vi "Add Test Suite - Without Id - Reports Error.vi"() -> ()   [LabVIEW 2013, in "JUnit XML Tests.lvlib" / "Test Suites.lvlib"]
uses:
  Test Suites.lvlib
  JUnit XML/Test Suite/Test Suite.lvclass/Test Suite.ctl
  JUnit XML/Test Suite/Write Timestamp.vi
  <vilib>/addons/_JKI Toolkits/Caraya/classes/Assert/Assert Error.vi
  <vilib>/addons/_JKI Toolkits/Caraya/classes/Test/Test.lvclass
  <vilib>/addons/_JKI Toolkits/Caraya/classes/Assert/Assert.lvclass
  JUnit XML/Test Suites/Test Suites.lvclass
  JUnit XML/Test Suite/Test Suite.lvclass
panel:
  out "error out":errorcluster
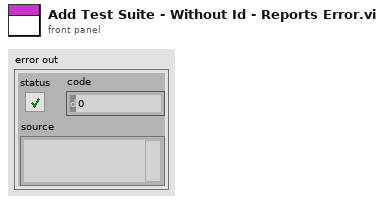
[diagram p1: front panel]
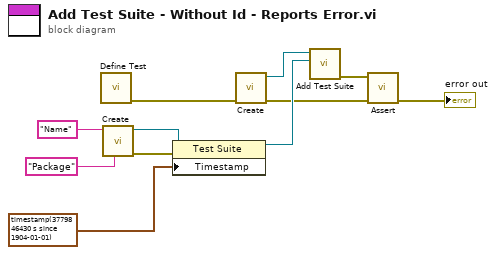
[diagram p0: block diagram]
diagram:
  n1 = call <vilib>:"Define Test.vi"() -> ("error out"=w4:errorcluster)  [unwired: 10 in, 1 out]
  n2 = call "Create.vi"("Package (\"\" = undefined)"="Package" ("Package (\"\" = undefined)"), "Name"="Name" ("Package")) -> ("error out"=w9:errorcluster, "Test Suite"=w8:refnum<class "Test Suite.lvclass">)  [unwired: 8 in]
  n3 = property class="Test Suite"(reference=w8, error in=w9, "Timestamp"=timestamp(3779846430.123 s since 1904-01-01)) -> (reference out=w5:refnum<class "Test Suite.lvclass">)  [unwired: 1 out]
  n4 = call "Create.vi"("error in (no error)"=w4) -> ("error out"=w2:errorcluster, "Test Suites"=w10:refnum<class "Test Suites.lvclass">)  [unwired: 9 in]
  n5 = call "Add Test Suite.vi"("Test Suite"=w5, "Test Suites in"=w10) -> ("error out"=w3:errorcluster)  [unwired: 8 in, 1 out]
  n6 = call-poly <vilib>:"Assert.vi"("error in (no error)"=w2, "Error?"=w3) -> ("error out"=→"error out":errorcluster)  [unwired: 8 in, 1 out]
